vi "wait.vi"(8 "error in":errorcluster, 9 "milliseconds to wait":u32, 11 "application reference in":refnum<vi>) -> (0 "error out":errorcluster, 3 "application reference out":refnum<vi>)   [LabVIEW 2014]
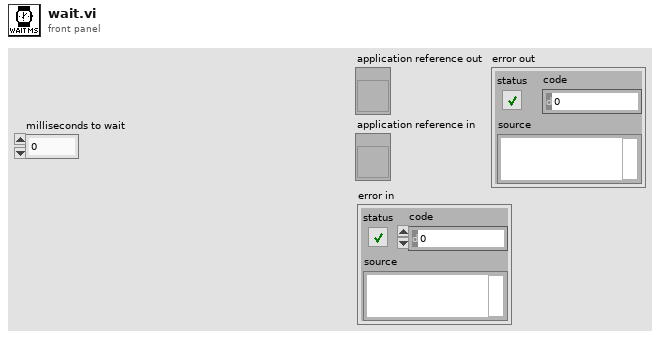
[diagram p1: front panel]
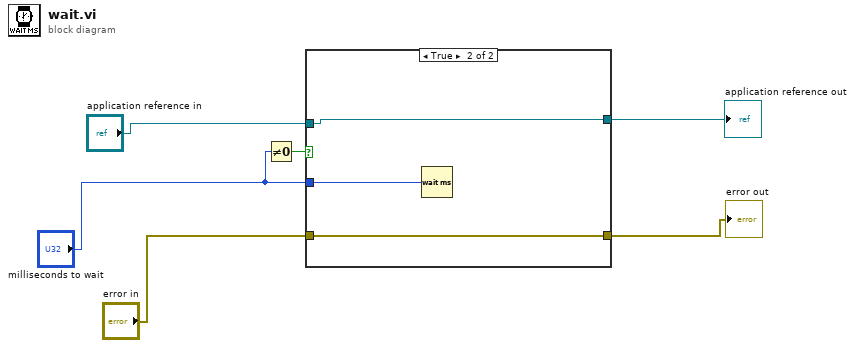
[diagram p0: block diagram]
diagram:
  n1 = Not Equal To 0?(x="milliseconds to wait") -> (x != 0?=w4:bool)
  n2 = case shown="True" w4 {
    tunnel: "application reference in" -> [w8 w11]
    tunnel: [w8 w11] -> w5
    tunnel: "milliseconds to wait" -> [_ w10]
    tunnel: "error in" -> [w7 w9]
    tunnel: [w7 w9] -> w1
    frame False {
    }
    frame True {
      n3 = Wait (ms)(milliseconds to wait=w10) -> ()  [unwired: 1 out]
    }
  }
  "application reference out" <- w5
  "error out" <- w1
